vi "Vector3_RotateYPR.vi"(1 "Yaw (degrees clockwise positive looking into z-axis)":dbl=-30.0, 2 "Pitch (degrees clockwise positive looking into x-axis)":dbl, 3 "Roll (degrees clockwise positive looking into y-axis)":dbl, 4 "Input Vector3":dbl[](array[numeric])=[0.0, -1.0, 0.0] format="%#.3g") -> (0 "Output Vector3":dbl[](array[numeric])=[0.49999999999999994, -0.8660254037844387, 0.0] format="%#.3g")   [LabVIEW 2010]
panel:
  # "IMPORTANT NOTE:\n\nThe order of the rotations is fixed as:\n\nYaw then Pitch then Roll.\n\nIf this order is not desired, then do each transformation\nseparately, setting the other angles to zero.\n\nXYZ axes are those defined for Enflo tunnel coordinate\nsystem!\n\nINPUT VECTOR MUST BE A DIRECTION VECTOR ONLY"
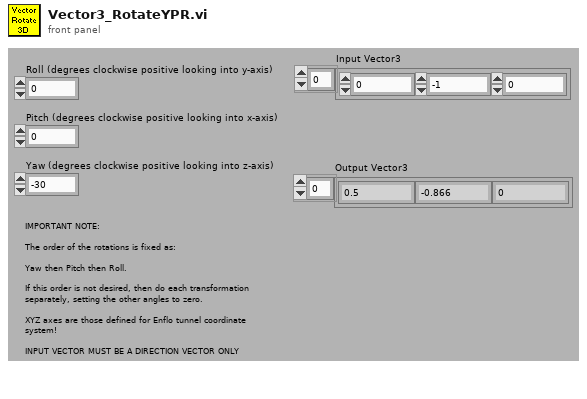
[diagram p1: front panel]
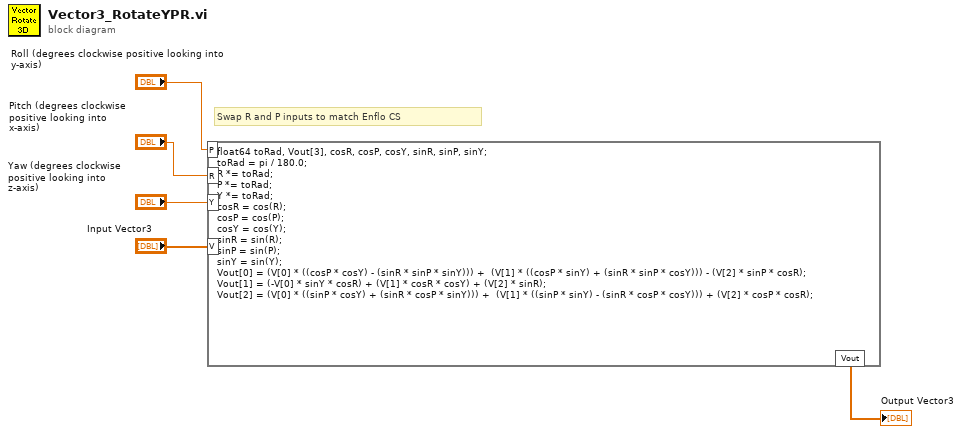
[diagram p0: block diagram]
diagram:
  # "Swap R and P inputs to match Enflo CS"
  n1 = formula code="float64 toRad, Vout[3], cosR, cosP, cosY, sinR, sinP, sinY;\ntoRad = pi / 180.0;\nR *= toRad;\nP *= toRad;\nY *= toRad;\ncosR = cos(R);\ncosP = cos(P);\ncosY = cos(Y);\nsinR = sin(R);\nsinP = sin(P);\nsinY = sin(Y);\nVout[0] = (V[0] * ((cosP * cosY) - (sinR * sinP * sinY))) +  (V[1] * ((cosP * sinY) + (sinR * sinP * cosY))) - (V[2] * sinP * cosR);\nVout[1] = (-V[0] * sinY * cosR) + (V[1] * cosR * cosY) + (V[2] * sinR);\nVout[2] = (V[0] * ((sinP * cosY) + (sinR * cosP * sinY))) +  (V[1] * ((sinP * sinY) - (sinR * cosP * cosY))) + (V[2] * cosP * cosR);"("P"="Roll (degrees clockwise positive looking into y-axis)", "R"="Pitch (degrees clockwise positive looking into x-axis)", "Y"="Yaw (degrees clockwise positive looking into z-axis)", "V"="Input Vector3") -> ("Vout"=→"Output Vector3":dbl[])
